vi "Systems_ReadConfig.vi"(4 "error in (no error)":errorcluster, 7 "configuration file path":path) -> (0 "error out":errorcluster, 2 "All Found?":bool)   [LabVIEW 2015]
uses:
  <vilib>/Utility/config.llb/NI_LVConfig.lvlib
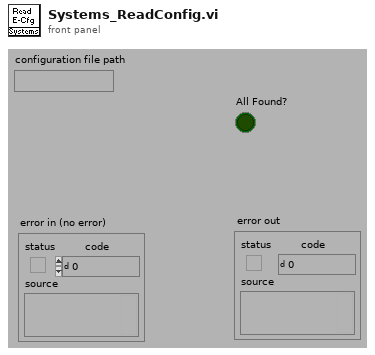
[diagram p1: front panel]
types:
  T1 = typedef "NI_LVConfig.lvlib/Config Data RefNum.ctl" = refnum<k1>
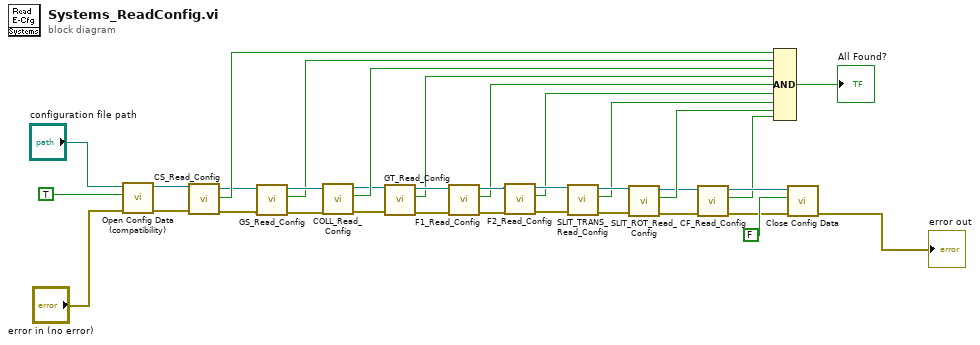
[diagram p0: block diagram]
diagram:
  n1 = call <vilib>:"Open Config Data (compatibility).vi"("error in (no error)"="error in (no error)", "create file if necessary (T)"=TRUE, "configuration file path"="configuration file path") -> ("error out"=w12:errorcluster, "refnum"=w13:T1)  [unwired: 6 in, 1 out]
  n2 = call "CS_Read_Config.vi"("error in (no error)"=w12, "Config refnum"=w13) -> ("error out"=w9:errorcluster, "All Found?"=w11:bool, "refnum out"=w10:T1)  [unwired: 3 in]
  n3 = call "GS_Read_Config.vi"("error in (no error)"=w9, "Config Refnum"=w10) -> ("error out"=w8:errorcluster, "All Found?"=w6:bool, "refnum out"=w7:T1)  [unwired: 3 in]
  n4 = call "COLL_Read_Config.vi"("error in (no error)"=w8, "Config Refnum"=w7) -> ("error out"=w15:errorcluster, "All Found?"=w24:bool, "refnum out"=w14:T1)  [unwired: 3 in]
  n5 = call "GT_Read_Config.vi"("error in (no error)"=w15, "Config Refnum"=w14) -> ("error out"=w34:errorcluster, "All Found?"=w23:bool, "refnum out"=w35:T1)  [unwired: 3 in]
  n6 = call "F1_Read_Config.vi"("error in (no error)"=w34, "Config Refnum"=w35) -> ("error out"=w32:errorcluster, "All Found?"=w22:bool, "refnum out"=w33:T1)  [unwired: 3 in]
  n7 = call "F2_Read_Config.vi"("error in (no error)"=w32, "Config Refnum"=w33) -> ("error out"=w30:errorcluster, "All Found?"=w21:bool, "refnum out"=w31:T1)  [unwired: 3 in]
  n8 = call "SLIT_TRANS_Read_Config.vi"("error in (no error)"=w30, "Config Refnum"=w31) -> ("error out"=w28:errorcluster, "All Found?"=w20:bool, "refnum out"=w29:T1)  [unwired: 3 in]
  n9 = call "SLIT_ROT_Read_Config.vi"("error in (no error)"=w28, "Config Refnum"=w29) -> ("error out"=w4:errorcluster, "All Found?"=w19:bool, "refnum out"=w5:T1)  [unwired: 3 in]
  n10 = call "CF_Read_Config.vi"("error in (no error)"=w4, "Config Refnum"=w5) -> ("error out"=w2:errorcluster, "All Found?"=w1:bool, "refnum out"=w3:T1)  [unwired: 3 in]
  n11 = Compound Arithmetic op=AND(w11, w6, w24, w23, w22, w21, w20, w19, w1) -> (→"All Found?":bool)
  n12 = call <vilib>:"Close Config Data.vi"("error in (no error)"=w2, "write file if changed (T)"=FALSE, "refnum"=w3) -> ("error out"=→"error out":errorcluster)  [unwired: 7 in, 1 out]
